vi "Get Employee Salary Info Names and Types.vi"(8 "错误输入（无错误）":errorcluster) -> (0 "错误输出":errorcluster, 1 "Colomn Types":variant[](array[variant]), 2 "Column Names":string[](array[string]))   [LabVIEW 2012]
uses:
  Custom Def/Salary Info.ctl
panel:
  in  "Salary Info":T1
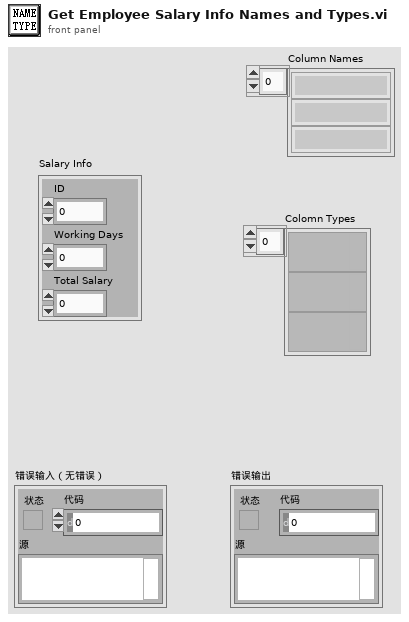
[diagram p1: front panel]
types:
  T1 = typedef "Salary Info.ctl" = cluster{"ID":u16, "Working Days":dbl, "Total Salary":dbl}
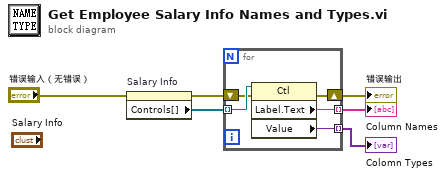
[diagram p0: block diagram]
diagram:
  n1 = property on="Salary Info" class="Clust (严格)"(error in="错误输入（无错误）") -> (error out=w1:errorcluster, "Controls[]"=w3:refnum<vi>[])  [unwired: 1 in, 1 out]
  n2 = for {
    tunnel: w3 -> [w11] mode=indexing
    tunnel: [w10] -> w5 mode=indexing
    tunnel: [w9] -> w4 mode=indexing
    shift-right: [w7] -> w6
    shift-left: w1 -> [w8]
    n3 = property class="Ctl"(reference=w11, error in=w8) -> (error out=w7:errorcluster, "Label.Text"=w10:string, "Value"=w9:variant)  [unwired: 1 out]
  }
  "错误输出" <- w6
  "Column Names" <- w5
  "Colomn Types" <- w4
